vi "create_grid.vi"(8 "Error In":errorcluster, 9 "Grid Constant":i32, 10 "Y Size":i32, 11 "X Size":i32) -> (0 "Error Out":errorcluster, 3 "Array":T1(array[cluster]))   [LabVIEW 2019]
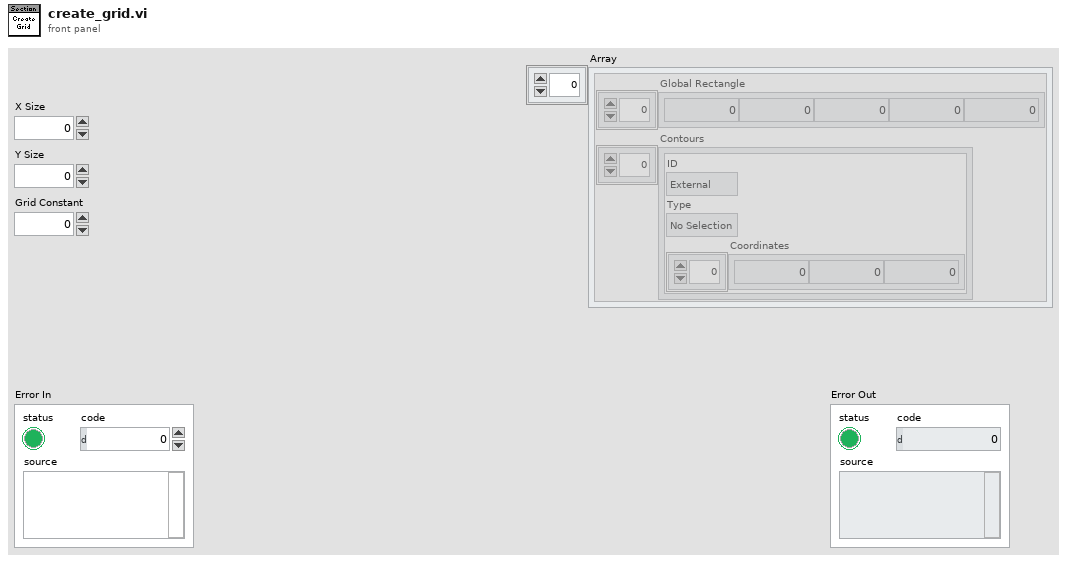
[diagram p1: front panel]
types:
  T1 = cluster{"Global Rectangle":i32[], "Contours":cluster{"ID":enum32{"External", "Internal"}, "Type":enum32{"No Selection", "Point", "Line", "Rectangle", "Oval", "Polygon", "Free", "Unused1", "Unused2", "Unused3", "Broken Line", "Free Hand Line"}, "Coordinates":i32[]}[]}[]
  T2 = cluster{"ID":enum32{"External", "Internal"}, "Type":enum32{"No Selection", "Point", "Line", "Rectangle", "Oval", "Polygon", "Free", "Unused1", "Unused2", "Unused3", "Broken Line", "Free Hand Line"}, "Coordinates":i32[]}
  T3 = cluster{"Global Rectangle":i32[], "Contours":cluster{"ID":enum32{"External", "Internal"}, "Type":enum32{"No Selection", "Point", "Line", "Rectangle", "Oval", "Polygon", "Free", "Unused1", "Unused2", "Unused3", "Broken Line", "Free Hand Line"}, "Coordinates":i32[]}[]}
  T4 = cluster{"ID":enum32{"External", "Internal"}, "Type":enum32{"No Selection", "Point", "Line", "Rectangle", "Oval", "Polygon", "Free", "Unused1", "Unused2", "Unused3", "Broken Line", "Free Hand Line"}, "Coordinates":i32[]}[]
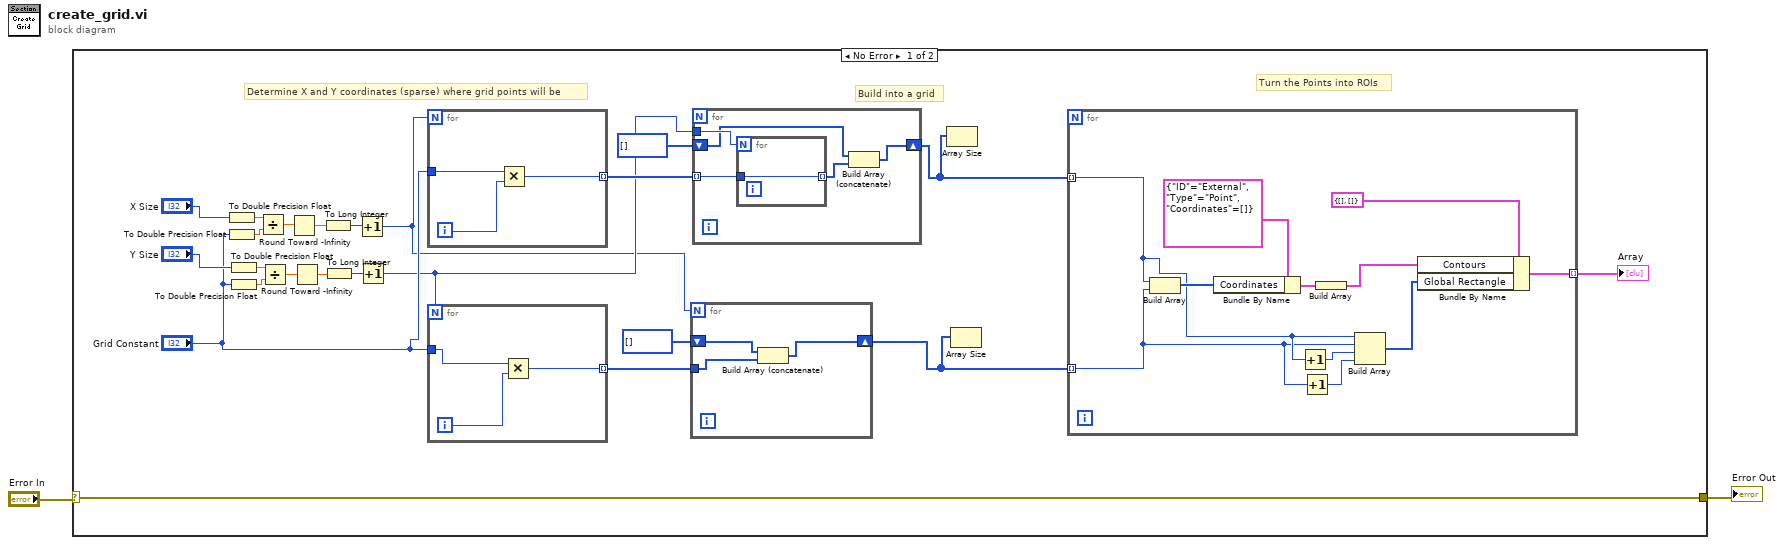
[diagram p0: block diagram]
diagram:
  n1 = case shown="No Error" "Error In" {
    selector: "Error In" -> [w11 w52]
    tunnel: [w11 w52] -> w1
    frame No Error {
      # "Build into a grid"
      # "Turn the Points into ROIs"
      # "Determine X and Y coordinates (sparse) where grid points will be"
      n2 = To Double Precision Float(number="X Size") -> (double precision float=w25:dbl)
      n3 = To Double Precision Float(number="Grid Constant") -> (double precision float=w24:dbl)
      n4 = To Double Precision Float(number="Y Size") -> (double precision float=w22:dbl)
      n5 = To Double Precision Float(number="Grid Constant") -> (double precision float=w23:dbl)
      n6 = Divide(x=w25, y=w24) -> (x/y=w19:dbl)
      n7 = Divide(x=w22, y=w23) -> (x/y=w18:dbl)
      n8 = Round Toward -Infinity(1:w19) -> (0:w16:dbl)
      n9 = Round Toward -Infinity(1:w18) -> (0:w17:dbl)
      n10 = To Long Integer(number=w16) -> (32bit integer=w13:i32)
      n11 = To Long Integer(number=w17) -> (32bit integer=w14:i32)
      n12 = Increment(x=w13) -> (x+1=w3:i32)
      n13 = Increment(x=w14) -> (x+1=w4:i32)
      n14 = for {
        N: w3 -> [_]
        tunnel: "Grid Constant" -> [w51]
        tunnel: [w49] -> w10 mode=indexing
        i -> [w50]
        n15 = Multiply(x=w51, y=w50) -> (x*y=w49:i32)
      }
      n16 = for {
        N: w4 -> [_]
        tunnel: "Grid Constant" -> [w47]
        tunnel: [w46] -> w7 mode=indexing
        i -> [w48]
        n17 = Multiply(x=w47, y=w48) -> (x*y=w46:i32)
      }
      n18 = for {
        N: w3 -> [_]
        tunnel: w7 -> [w27]
        shift-right: [w26] -> w5
        shift-left: i32[] [] -> [w28]
        n19 = Build Array (concatenate)(w28, w27) -> (w26:i32[])
      }
      n20 = for {
        tunnel: w10 -> [w33] mode=indexing
        shift-right: [w29] -> w6
        shift-left: i32[] [] -> [w30]
        tunnel: w4 -> [w32]
        n21 = for {
          N: w32 -> [_]
          tunnel: w33 -> [w34]
          tunnel: [w34] -> w31 mode=indexing
        }
        n22 = Build Array (concatenate)(w30, w31) -> (w29:i32[])
      }
      n23 = Array Size(array=w6) -> ()  [unwired: 1 out]
      n24 = Array Size(array=w5) -> ()  [unwired: 1 out]
      n25 = for {
        tunnel: w6 -> [w38] mode=indexing
        tunnel: w5 -> [w37] mode=indexing
        tunnel: [w35] -> w12 mode=indexing
        n26 = Build Array(w38, w37) -> (w43:i32[])
        n27 = Bundle By Name(cluster=T2 {"ID"=enum."External", "Type"=enum."Point", "Coordinates"=[]}, "Coordinates"=w43) -> (w42:T2)
        n28 = Increment(x=w38) -> (x+1=w36:i32)
        n29 = Increment(x=w37) -> (x+1=w39:i32)
        n30 = Build Array(w42) -> (w41:T4)
        n31 = Build Array(w38, w37, w36, w39) -> (w40:i32[])
        n32 = Bundle By Name(cluster=T3 {"Global Rectangle"=[], "Contours"=[]}, "Contours"=w41, "Global Rectangle"=w40) -> (w35:T3)
      }
      "Array" <- w12
    }
    frame Error {
    }
  }
  "Error Out" <- w1
